vi "Progress Bar FGV.vi"(6 "Progress Refnum":refnum<vi>, 7 "Prog Bar States":T1, 8 "error in (no error)":errorcluster, 11 "Total Size":i32) -> (0 "error out":errorcluster)   [LabVIEW 2013]
uses:
  Progress bar enum.ctl
panel:
  out "x*y":dbl
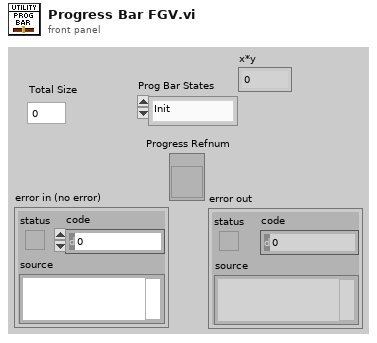
[diagram p1: front panel]
types:
  T1 = typedef "Progress bar enum.ctl" = enum16{"Init", "Increment"}
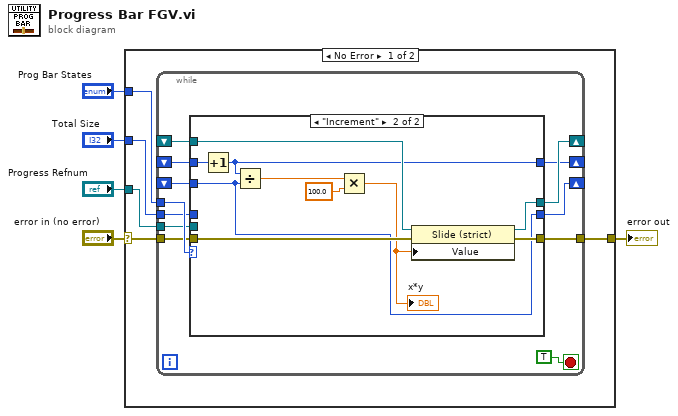
[diagram p0: block diagram]
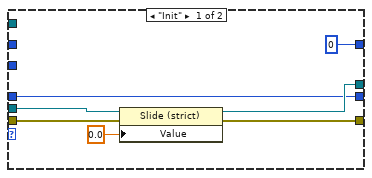
[diagram p2: hidden frame]
diagram:
  n1 = case shown="No Error" "error in (no error)" {
    selector: "error in (no error)" -> [w8 w40]
    tunnel: [w7 w40] -> w4
    tunnel: "Progress Refnum" -> [w10 _]
    tunnel: "Prog Bar States" -> [w9 _]
    tunnel: "Total Size" -> [w6 _]
    frame No Error {
      n2 = while {
        tunnel: w10 -> [w19]
        tunnel: w9 -> [w21]
        shift-right: [w20] -> _
        shift-left: _ -> [w16]
        tunnel: w8 -> [w18]
        tunnel: [w17] -> w7
        shift-right: [w14] -> _
        shift-left: _ -> [w15]
        shift-right: [w12] -> _
        shift-left: _ -> [w13]
        tunnel: w6 -> [w11]
        stop <- TRUE stop-if-true
        n3 = case shown="\"Increment\"" w21 {
          tunnel: [w28 w39] -> w20
          tunnel: w19 -> [w29 _]
          tunnel: w18 -> [w26 w38]
          tunnel: [w25 w37] -> w17
          tunnel: w16 -> [_ w36]
          tunnel: w15 -> [_ w35]
          tunnel: [0 ("File Count") w30] -> w14
          tunnel: w13 -> [_ w34]
          tunnel: [w23 w34] -> w12
          tunnel: w11 -> [w23 _]
          frame "Init" {
            n4 = property class="Slide (strict)"(reference=w29, error in=w26, "Value"=0.0) -> (reference out=w28:refnum<vi>, error out=w25:errorcluster)
          }
          frame "Increment" {
            n5 = Increment(x=w35) -> (x+1=w30:i32)
            n6 = Divide(x=w30, y=w34) -> (x/y=w33:dbl)
            n7 = Multiply(x=w33, y=100.0) -> (x*y=w31:dbl)
            "x*y" <- w31
            n8 = property class="Slide (strict)"(reference=w36, error in=w38, "Value"=w31) -> (reference out=w39:refnum<vi>, error out=w37:errorcluster)
          }
        }
      }
    }
    frame Error {
    }
  }
  "error out" <- w4
